vi "Keithley 3390 Standard Waveform.vi"() -> ()   [LabVIEW 2017]
doc: "This example shows how to configure and output a standard waveform."
uses:
  Keithley 3390.lvlib
  Public/Configure/Configure Waveform (Sine).vi
panel:
  in  "DC Offset (0.00 V)":dbl
  in  "Frequency (1000 Hz)":dbl=1000.0
  in  "Amplitude (1.0 Vpp)":dbl=1.0
  in  "VISA resource name":refnum<visa-resource-name>
  # "(c) 2008 Keithley Instruments, Inc.  ALL RIGHTS RESERVED."
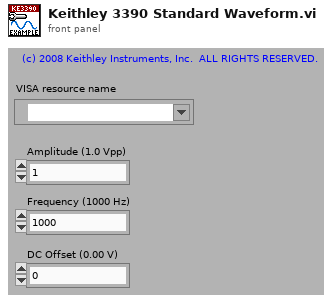
[diagram p1: front panel]
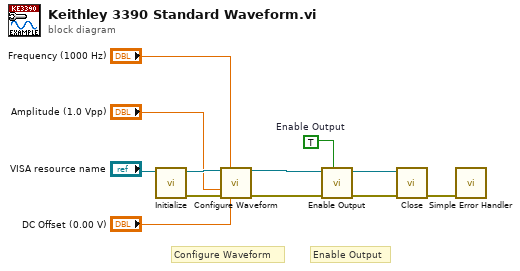
[diagram p0: block diagram]
diagram:
  w1 = TRUE  # Enable Output
  # "Enable Output"
  # "Configure Waveform"
  n1 = call "Initialize.vi"("VISA resource name"="VISA resource name") -> ("error out"=w10:errorcluster, "VISA resource name out"=w11:refnum<visa-resource-name>)  [unwired: 9 in]
  n2 = call-poly "Configure Waveform.vi"("VISA resource name"=w11, "Frequency (1000 Hz)"="Frequency (1000 Hz)", "Amplitude (1.0 Vpp)"="Amplitude (1.0 Vpp)", "error in (no error)"=w10, "DC Offset (0.00 V)"="DC Offset (0.00 V)") -> ("VISA resource name out"=w6:refnum<visa-resource-name>, "error out"=w5:errorcluster)  [unwired: 9 in]
  n3 = call "Enable Output.vi"("Enable Output (T: Enable)"=w1, "error in (no error)"=w5, "VISA resource name"=w6) -> ("error out"=w3:errorcluster, "VISA resource name out"=w4:refnum<visa-resource-name>)  [unwired: 7 in]
  n4 = call "Close.vi"("error in (no error)"=w3, "VISA resource name"=w4) -> ("error out"=w7:errorcluster)  [unwired: 9 in]
  n5 = call <vilib>:"Simple Error Handler.vi"("error in (no error)"=w7) -> ()  [unwired: 4 in, 5 out]
